vi "Single-Loop Queued State Machine.vi"() -> ()   [LabVIEW 2020]
uses:
  VIPackages/Custom Packages/Source LV2020-32b/SM Templates/StateMachine - AppData--cluster.ctl
panel:
  in  "Exit":bool
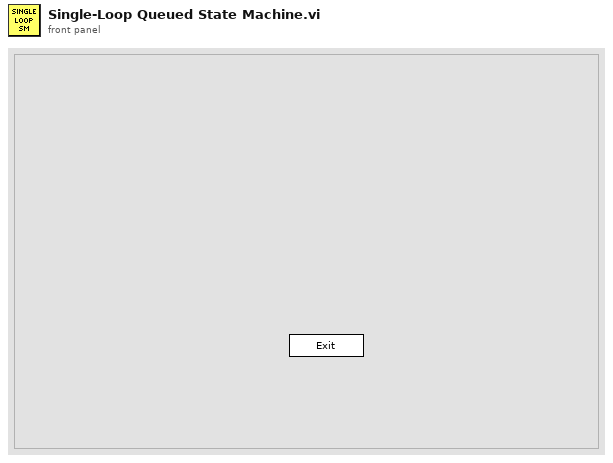
[diagram p1: front panel]
types:
  T1 = typedef "StateMachine - AppData--cluster.ctl" = cluster{"Core":cluster{"Current VI Reference":refnum<vi>, "Close Panel on Exit?":bool}, "Your Boolean data":bool, "Your string data":string}
  T2 = enum32{"invalid app kind", "Development System", "Run Time System", "Student Edition", "Embedded LabVIEW", "Evaluation", "Custom"}
  T3 = enum32{"Invalid", "Standard", "Closed", "Hidden", "Minimized", "Maximized"}
  T4 = cluster{"Current VI Reference":refnum<vi>, "Close Panel on Exit?":bool}
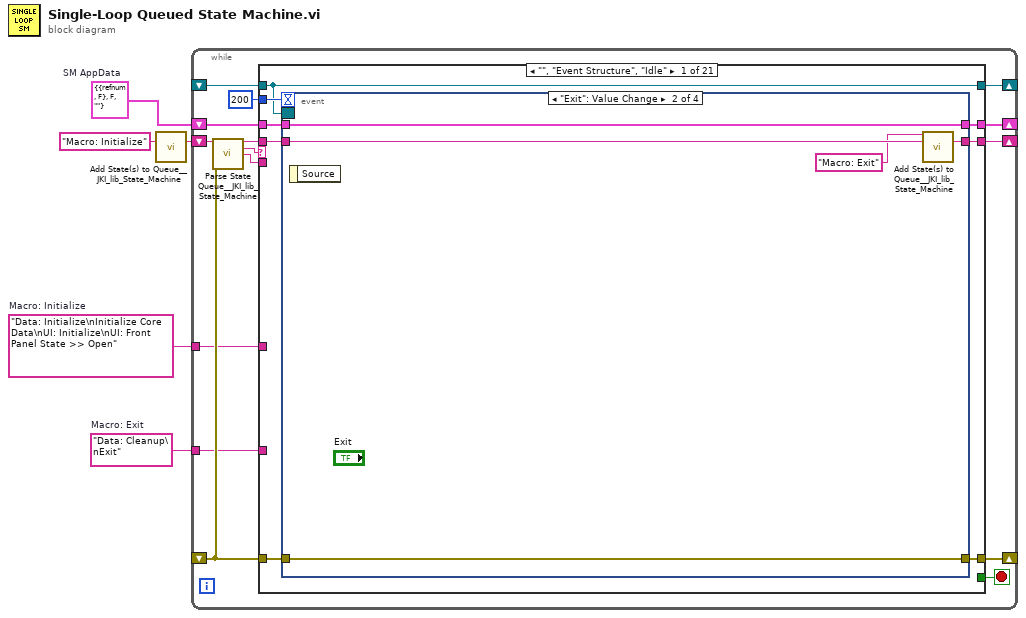
[diagram p0: block diagram]
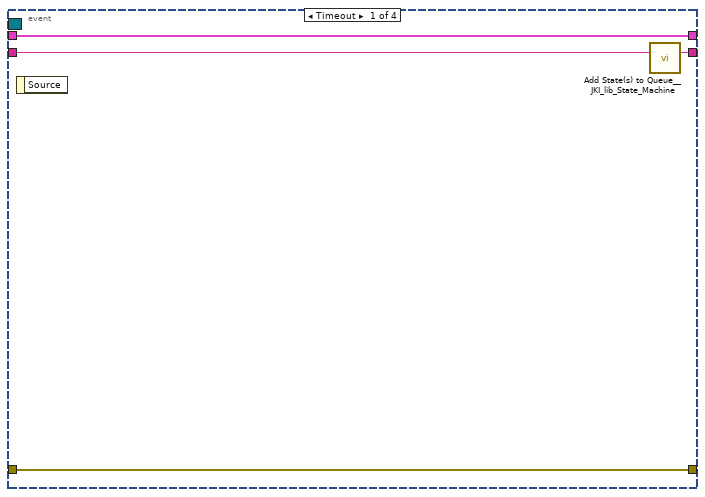
[diagram p2: hidden frame]
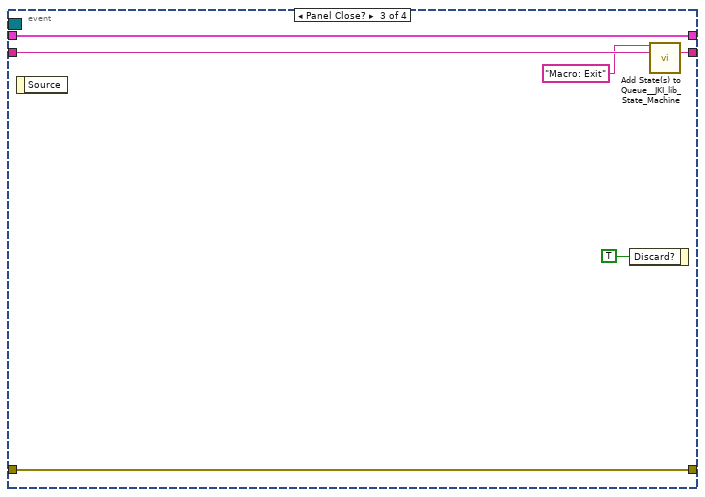
[diagram p3: hidden frame]
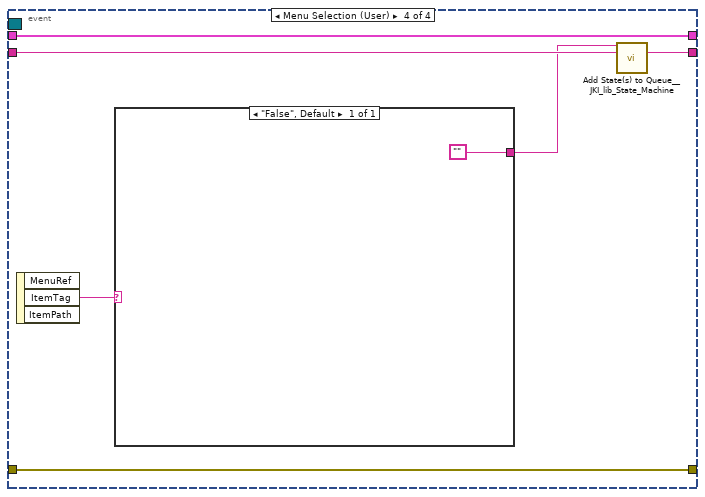
[diagram p4: hidden frame]
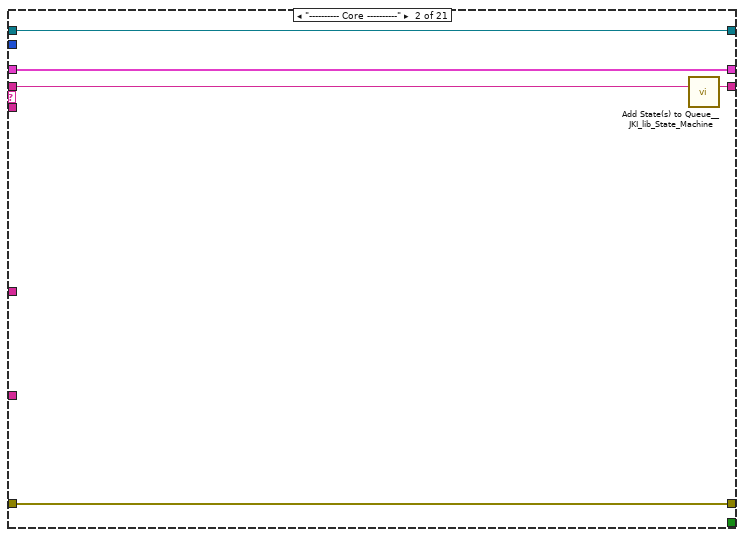
[diagram p5: hidden frame]
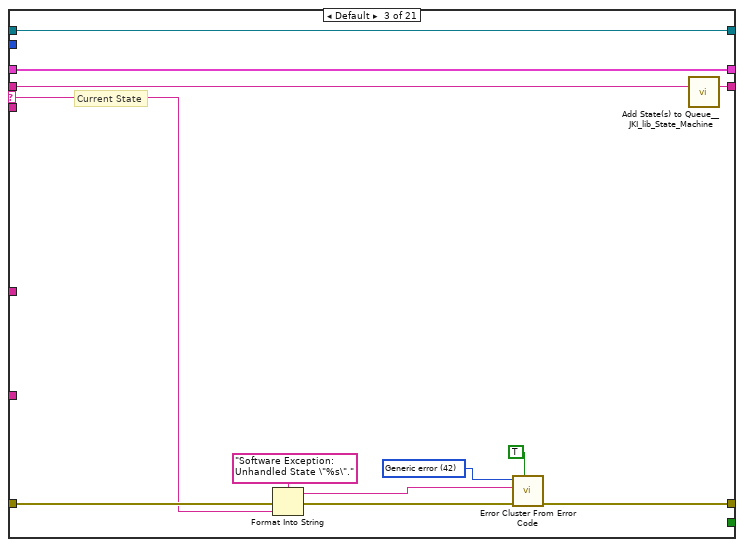
[diagram p6: hidden frame]
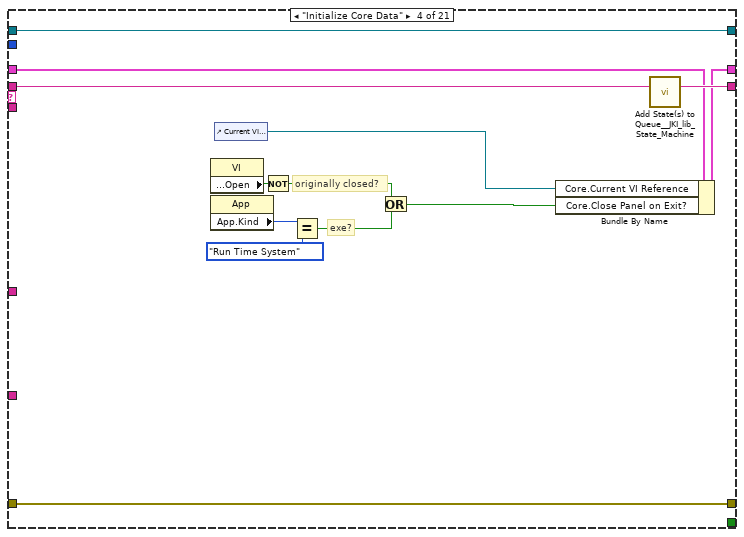
[diagram p7: hidden frame]
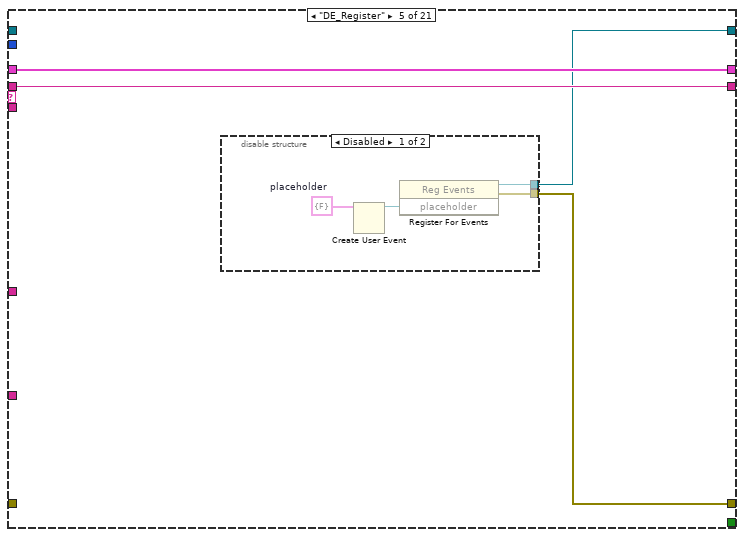
[diagram p8: hidden frame]
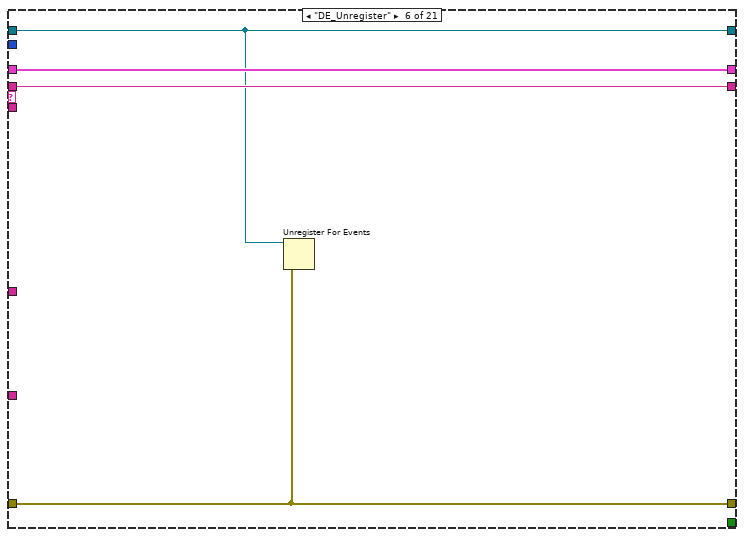
[diagram p10: hidden frame]
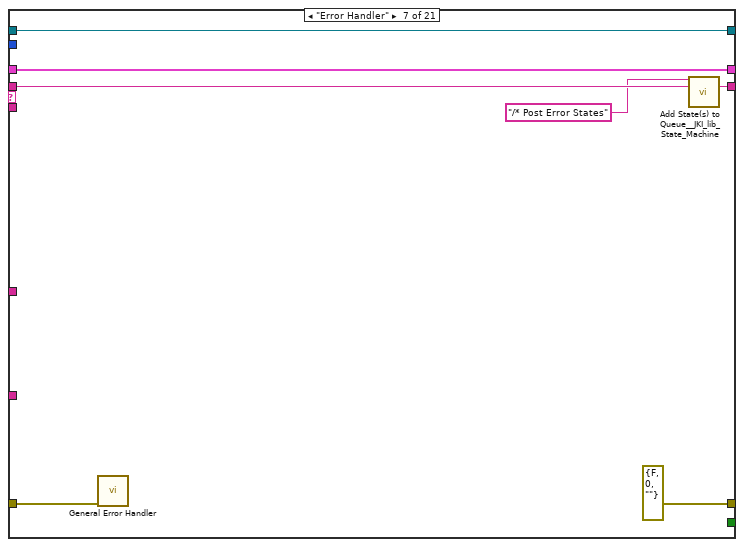
[diagram p11: hidden frame]
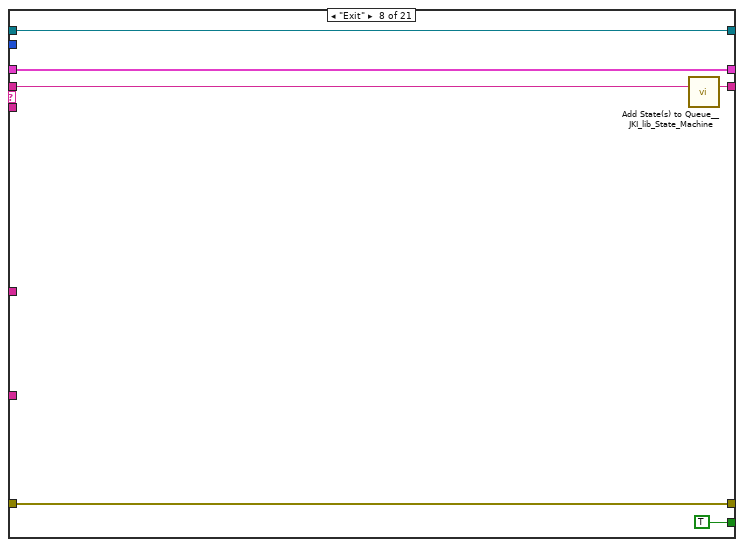
[diagram p12: hidden frame]
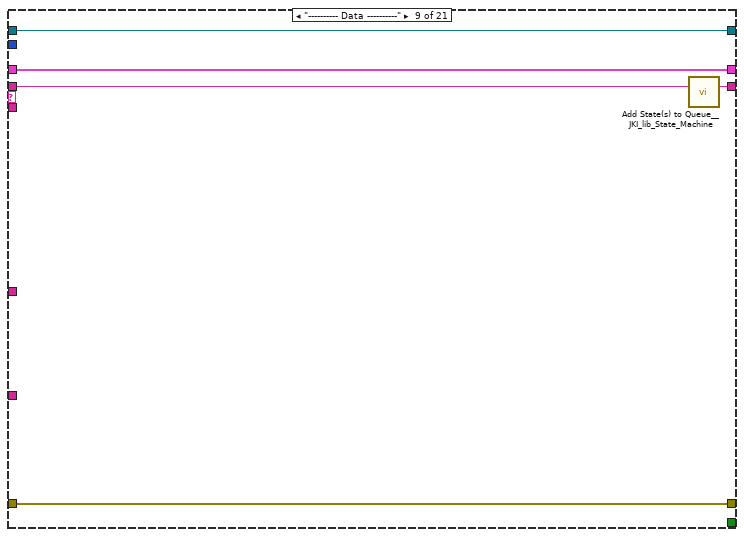
[diagram p13: hidden frame]
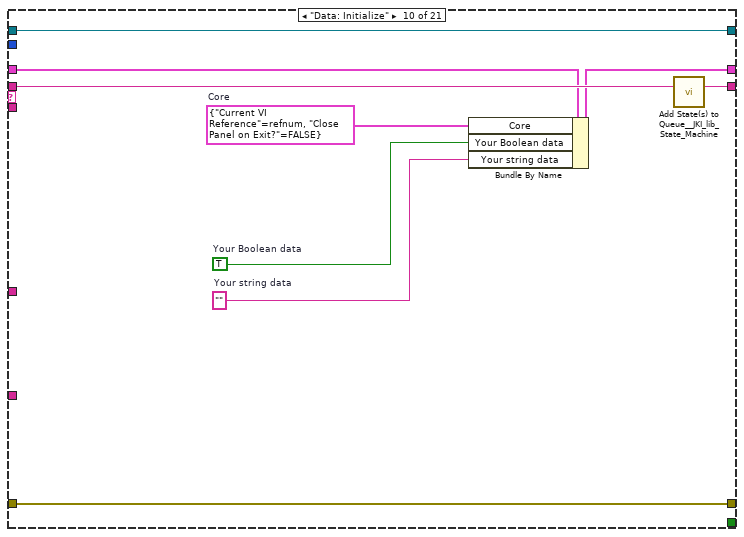
[diagram p14: hidden frame]
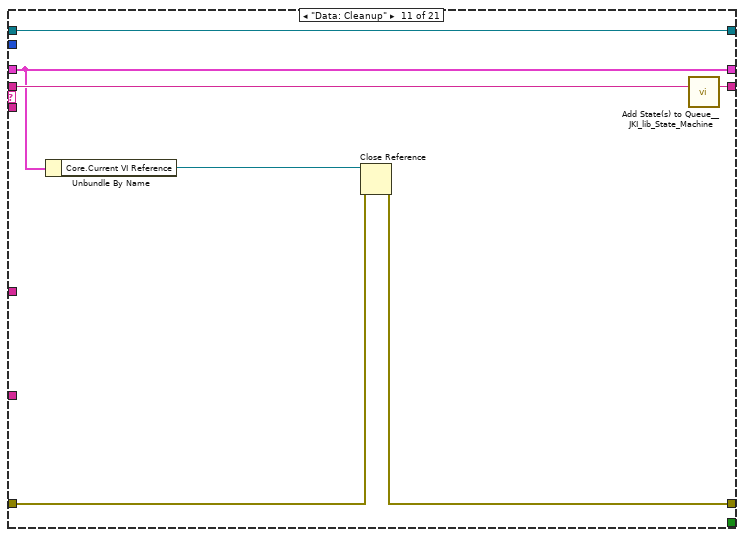
[diagram p15: hidden frame]
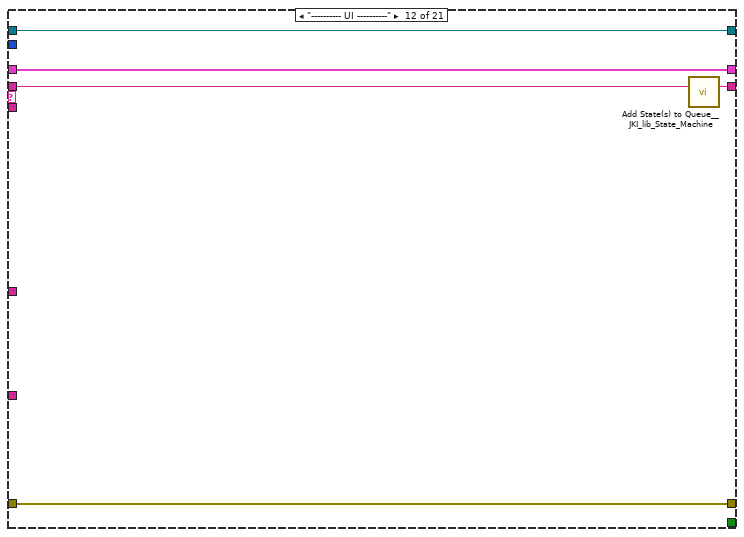
[diagram p16: hidden frame]
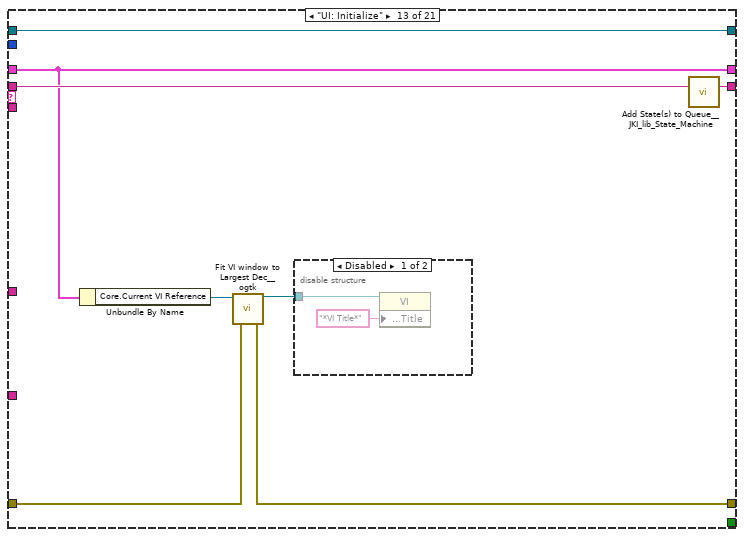
[diagram p17: hidden frame]
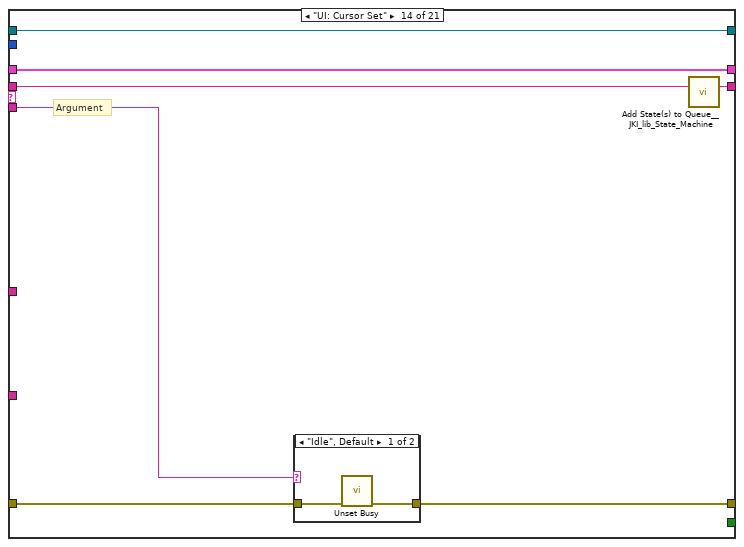
[diagram p19: hidden frame]
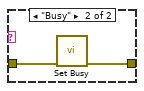
[diagram p20: hidden frame]
diagram:
  w1 = "Data: Cleanup\nExit"  # Macro: Exit
  w2 = "Data: Initialize\nInitialize Core Data\nUI: Initialize\nUI: Front Panel State >> Open"  # Macro: Initialize
  w3 = T1 {"Core"={"Current VI Reference"=refnum, "Close Panel on Exit?"=FALSE}, "Your Boolean data"=FALSE, "Your string data"=""}  # SM AppData
  n1 = call <vilib>:"Add State(s) to Queue__JKI_lib_State_Machine.vi"("State(s) in (\"\")"="Macro: Initialize") -> ("States Out"=w5:string)  [unwired: 14 in]
  n2 = while {
    shift-right: [w13] -> _
    shift-left: w3 -> [w12]
    shift-right: [w16] -> _
    shift-left: _ -> [w11]
    shift-right: [w15] -> _
    shift-left: w5 -> [w17]
    shift-right: [w10] -> _
    shift-left: _ -> [w9]
    tunnel: w2 -> [w7]
    tunnel: w1 -> [w6]
    stop <- w14 stop-if-true
    n3 = call <vilib>:"Parse State Queue__JKI_lib_State_Machine.vi"("State Queue"=w17, "Error In (no error)"=w11) -> ("Remaining States"=w19:string, "Current State"=w20:string, "Arguments"=w18:string)  [unwired: 11 in]
    n4 = case shown="\"\", \"Event Structure\", \"Idle\"" w20 {
      selector: w20 -> [_ _ w57 _ _ _ _ _ _ _ _ _ _ _ _ _ _ _ _ _ _]
      tunnel: w19 -> [w28 w55 w61 w80 w84 w92 w99 w105 w110 w119 w126 w131 w139 w148 w160 w187 w193 w204 w209 w220 w225]
      tunnel: w18 -> [_ _ _ _ _ _ _ _ _ _ _ _ _ w143 w154 _ _ _ _ w210 _]
      tunnel: w12 -> [w26 w52 w59 w71 w83 w91 w96 w103 w107 w113 w121 w128 w134 w146 w156 w184 w190 w201 w206 w218 w222]
      tunnel: [w25 w53 w63 w77 w81 w89 errorcluster {"status"=FALSE, "code"=0, "source"=""} ("error out") w102 w108 w117 w122 w129 w135 w144 w157 w185 w191 w202 w207 w211 w223] -> w16
      tunnel: w11 -> [w24 w53 w62 w77 _ w89 w95 w102 w108 w117 w123 w129 w136 w145 w158 w185 w191 w202 w207 w212 w223]
      tunnel: [w27 w54 w60 w79 w84 w92 w98 w104 w109 w118 w125 w130 w138 w147 w159 w186 w192 w203 w208 w219 w224] -> w15
      tunnel: [_ _ _ _ _ _ _ TRUE _ _ _ _ _ _ _ _ _ _ _ _ _] -> w14
      tunnel: [w23 w52 w59 w78 w83 w91 w96 w103 w107 w112 w121 w128 w134 w146 w156 w184 w190 w201 w206 w218 w222] -> w13
      tunnel: [w21 w51 w56 w68 w82 w90 w93 w100 w106 w111 w120 w127 w137 w142 w153 w183 w189 w195 w205 w217 w221] -> w10
      tunnel: w9 -> [w21 w51 w56 w68 _ w90 w93 w100 w106 w111 w120 w127 w137 w142 w153 w183 w189 w195 w205 w217 w221]
      tunnel: 200 ("Timeout") -> [w22 _ _ _ _ _ _ _ _ _ _ _ _ _ _ _ _ _ _ _ _]
      tunnel: w7 -> [_ _ _ _ _ _ _ _ _ _ _ _ _ _ _ _ w188 _ _ _ _]
      tunnel: w6 -> [_ _ _ _ _ _ _ _ _ _ _ _ _ _ _ _ _ w194 _ _ _]
      frame "", "Event Structure", "Idle" {
        n5 = event shown="[1] \"Exit\": Value Change" {
          selector: w21 -> [_ _ _ _]
          dyn-events: _ -> [_ _ _ _]
          timeout: w22 -> [_ _ _ _]
          tunnel: w28 -> [w32 w37 w43 w46]
          tunnel: [w31 w36 w42 w45] -> w27
          tunnel: w26 -> [w29 w34 w40 w48]
          tunnel: [w30 w35 w41 w49] -> w25
          tunnel: w24 -> [w30 w35 w41 w49]
          tunnel: [w29 w34 w40 w48] -> w23
          event Timeout {
            n6 = event-data() -> ()  [unwired: 1 in, 1 out]
            n7 = call <vilib>:"Add State(s) to Queue__JKI_lib_State_Machine.vi"("State(s) in (\"\")"=w32) -> ("States Out"=w31:string)  [unwired: 14 in]
          }
          event "Exit": Value Change {
            n8 = event-data() -> ()  [unwired: 1 in, 1 out]
            n9 = call <vilib>:"Add State(s) to Queue__JKI_lib_State_Machine.vi"("State(s) in Front (\"\")"="Macro: Exit", "State(s) in (\"\")"=w37) -> ("States Out"=w36:string)  [unwired: 13 in]
          }
          event Panel Close? {
            n10 = event-data() -> ()  [unwired: 1 in, 1 out]
            n11 = event-data("Discard?"=TRUE) -> ()  [unwired: 1 in, 1 out]
            n12 = call <vilib>:"Add State(s) to Queue__JKI_lib_State_Machine.vi"("State(s) in Front (\"\")"="Macro: Exit", "State(s) in (\"\")"=w43) -> ("States Out"=w42:string)  [unwired: 13 in]
          }
          event Menu Selection (User) {
            n13 = event-data() -> ("ItemTag"=w47:string)  [unwired: 1 in, 2 out]
            n14 = case shown="\"False\", Default" w47 {
              tunnel: [""] -> w44
              frame "False", Default {
              }
            }
            n15 = call <vilib>:"Add State(s) to Queue__JKI_lib_State_Machine.vi"("State(s) in Front (\"\")"=w44, "State(s) in (\"\")"=w46) -> ("States Out"=w45:string)  [unwired: 13 in]
          }
        }
      }
      frame "---------- Core ----------" {
        n16 = call <vilib>:"Add State(s) to Queue__JKI_lib_State_Machine.vi"("State(s) in (\"\")"=w55) -> ("States Out"=w54:string)  [unwired: 14 in]
      }
      frame Default {
        w66 = 42 items=["No error", "Argument error", "Memory is full", "Out of zone", "End of file", "File already open", "Generic file I/O error", "File not found", "File permission error", "Disk is full", "Duplicate path", "Too many files open", "System feature not enabled", "Resource file not found", "Cannot add resource", "Resource not found", "Image not found", "Image memory error", "Pen does not exist", "Config type invalid", "Config token not found", "Config parse error", "Config memory error", "Bad external code format", "Bad external code offset", "External code not present", "Null window", "Destroy window error", "Null menu", "Print aborted", "Bad print record", "Print driver error", "Windows error during printing", "Memory error during printing", "Print dialog error", "Generic print error", "Invalid device refnum", "Device not found", "Device parameter error", "Device unit error", "Cannot open device", "Device call aborted", "Generic error", "Cancelled by user", "Object ID too low", "Object ID too high", "Object not in heap", "Unknown heap", "Unknown object (invalid DefProc)", "Unknown object (DefProc not in table)", "Message out of range", "Invalid (null) method", "Unknown message", "Manager call not supported", "Bad address", "Network operation in progress", "Network operation timed out", "Connection is busy", "Network attribute not supported", "Network error", "Address in use", "System out of memory", "Connection aborted", "Connection refused", "Not connected", "Already connected", "Connection closed", "Initialization error (interapplication manager)", "Bad occurrence", "Wait on unbound occurrence handler", "Occurrence queue overflow", "Datalog type conflict", "Unused", "Unrecognized type (interapplication manager)", "Memory corrupt", "Failed to make temporary DLL", "Old CIN version", "Drag socket not found", "Failed to load drop-object", "Failed to register OLE object", "Failed to release OLE object", "Format specifier type mismatch", "Unknown format specifier", "Too few format specifiers", "Too many format specifiers", "Scan failed", "Newer CIN version", "Error converting to variant", "Runtime menu error", "Password tampered", "Variant attribute not found", "Incompatible variant data type", "Event data is not available", "Event Store is not present", "Occurrence is not found", "Event Queue is not created", "Event info is not available", "Refnum passed is NULL", "Error retrieving Class GUID", "Error retrieving CoClass GUID", "Error retrieving TypeLib GUID.", "Bad built application magic bytes.", "Specific driver is different from the specific driver associated with the Logical Name.", "There is no session opened to the class driver.", "Max Error", "MAX - Error with config objects", "MAX - Error loading configuration", "MAX - Group not supported"]
        # "Current State"
        n17 = Format Into String(format string="Software Exception: Unhandled State \"%s\"." ("message"), error in=w62, w57) -> (resulting string=w65:string, error out=w64:errorcluster)  [unwired: 1 in]
        n18 = call <vilib>:"Error Cluster From Error Code.vi"("show call chain? (False)"=TRUE, "error in (no error)"=w64, "error message (\"\")"=w65, "error code (0)"=w66) -> ("error out"=w63:errorcluster)  [unwired: 5 in]
        n19 = call <vilib>:"Add State(s) to Queue__JKI_lib_State_Machine.vi"("State(s) in (\"\")"=w61) -> ("States Out"=w60:string)  [unwired: 14 in]
      }
      frame "Initialize Core Data" {
        # "originally closed?"
        # "exe?"
        n20 = property class="VI"() -> ("Front Panel.Open"=w76:bool)  [unwired: 2 in, 2 out]
        n21 = property class="App"() -> ("App.Kind"=w75:T2)  [unwired: 2 in, 2 out]
        n22 = control-ref of="Current VI Reference"() -> (w69:refnum<vi>)
        n23 = Not(x=w76) -> (.not. x?=w73:bool)
        n24 = Equal?(x=w75, y=T2."Run Time System" ("Application:Kind")) -> (x = y?=w72:bool)
        n25 = Or(x=w73, y=w72) -> (x .or. y?=w70:bool)
        n26 = Bundle By Name(cluster=w71, "Core.Current VI Reference"=w69, "Core.Close Panel on Exit?"=w70) -> (w78:T1)
        n27 = call <vilib>:"Add State(s) to Queue__JKI_lib_State_Machine.vi"("State(s) in (\"\")"=w80) -> ("States Out"=w79:string)  [unwired: 14 in]
      }
      frame "DE_Register" {
        n28 = disable-structure shown="Disabled" {
          disable-tunnel: [w88 _] -> w82
          disable-tunnel: [w87 _] -> w81
          frame Disabled {
            w86 = cluster{bool} {FALSE}  # placeholder
            n29 = Create User Event(user event datatype=w86) -> (user event=w85:refnum<user-event>)  [unwired: 1 in, 1 out]
            n30 = register-events(w85) -> (reference out=w88:refnum<event-registration>, error out=w87:errorcluster)  [unwired: 2 in]
          }
          frame Enabled {
          }
        }
      }
      frame "DE_Unregister" {
        n31 = Unregister For Events(event registration refnum=w90, error in=w89) -> ()  [unwired: 1 out]
      }
      frame "Error Handler" {
        n32 = call <vilib>:"General Error Handler.vi"("error in (no error)"=w95) -> ()  [unwired: 10 in, 5 out]
        n33 = call <vilib>:"Add State(s) to Queue__JKI_lib_State_Machine.vi"("State(s) in Front (\"\")"="/* Post Error States", "State(s) in (\"\")"=w99) -> ("States Out"=w98:string)  [unwired: 13 in]
      }
      frame "Exit" {
        n34 = call <vilib>:"Add State(s) to Queue__JKI_lib_State_Machine.vi"("State(s) in (\"\")"=w105) -> ("States Out"=w104:string)  [unwired: 14 in]
      }
      frame "---------- Data ----------" {
        n35 = call <vilib>:"Add State(s) to Queue__JKI_lib_State_Machine.vi"("State(s) in (\"\")"=w110) -> ("States Out"=w109:string)  [unwired: 14 in]
      }
      frame "Data: Initialize" {
        w114 = T4 {"Current VI Reference"=refnum, "Close Panel on Exit?"=FALSE}  # Core
        w116 = TRUE  # Your Boolean data
        w115 = ""  # Your string data
        n36 = Bundle By Name(cluster=w113, "Core"=w114, "Your Boolean data"=w116, "Your string data"=w115) -> (w112:T1)
        n37 = call <vilib>:"Add State(s) to Queue__JKI_lib_State_Machine.vi"("State(s) in (\"\")"=w119) -> ("States Out"=w118:string)  [unwired: 14 in]
      }
      frame "Data: Cleanup" {
        n38 = Unbundle By Name(w121) -> ("Core.Current VI Reference"=w124:refnum<vi>)
        n39 = Close Reference(reference=w124, error in (no error)=w123) -> (error out=w122:errorcluster)
        n40 = call <vilib>:"Add State(s) to Queue__JKI_lib_State_Machine.vi"("State(s) in (\"\")"=w126) -> ("States Out"=w125:string)  [unwired: 14 in]
      }
      frame "---------- UI ----------" {
        n41 = call <vilib>:"Add State(s) to Queue__JKI_lib_State_Machine.vi"("State(s) in (\"\")"=w131) -> ("States Out"=w130:string)  [unwired: 14 in]
      }
      frame "UI: Initialize" {
        n42 = Unbundle By Name(w134) -> ("Core.Current VI Reference"=w133:refnum<vi>)
        n43 = call <userlib>:"Fit VI window to Largest Dec__ogtk.vi"("error in (no error)"=w136, "VI Ref (calling VI)"=w133) -> ("error out"=w135:errorcluster, "dup VI Ref"=w132:refnum<vi>)  [unwired: 4 in]
        n44 = disable-structure shown="Disabled" {
          disable-tunnel: w132 -> [w141 _]
          frame Disabled {
            n45 = property class="VI"(reference=w141, "Front Panel.Title"="*VI Title*" ("Front Panel Window:Title")) -> ()  [unwired: 1 in, 2 out]
          }
          frame Enabled {
          }
        }
        n46 = call <vilib>:"Add State(s) to Queue__JKI_lib_State_Machine.vi"("State(s) in (\"\")"=w139) -> ("States Out"=w138:string)  [unwired: 14 in]
      }
      frame "UI: Cursor Set" {
        # "Argument"
        n47 = case shown="\"Idle\", Default" w143 {
          tunnel: w145 -> [w150 w152]
          tunnel: [w149 w151] -> w144
          frame "Idle", Default {
            n48 = call <vilib>:"Unset Busy.vi"("error in (no error)"=w150) -> ("error out"=w149:errorcluster)  [unwired: 10 in]
          }
          frame "Busy" {
            n49 = call <vilib>:"Set Busy.vi"("error in (no error)"=w152) -> ("error out"=w151:errorcluster)  [unwired: 9 in, 1 out]
          }
        }
        n50 = call <vilib>:"Add State(s) to Queue__JKI_lib_State_Machine.vi"("State(s) in (\"\")"=w148) -> ("States Out"=w147:string)  [unwired: 14 in]
      }
      frame "UI: Front Panel State" {
        # "Argument"
        n51 = Unbundle By Name(w156) -> ("Core.Current VI Reference"=w155:refnum<vi>)
        n52 = case shown="\"Close\"" w154 {
          tunnel: w158 -> [w164 w177]
          tunnel: [w166 w178] -> w157
          tunnel: w155 -> [w165 w175]
          frame "Open", Default {
            n53 = property class="VI"(reference=w165, error in=w164) -> (reference out=w162:refnum<vi>, error out=w163:errorcluster, "Front Panel.Open"=w161:bool)
            n54 = case shown="False" w161 {
              tunnel: [w169 w172] -> w166
              tunnel: w163 -> [w168 w172]
              tunnel: w162 -> [w167 _]
              frame False {
                n55 = invoke class="VI" method="FP.Open"(reference=w167, error in=w168, "Activate"=TRUE, "State"=T3."Standard") -> (error out=w169:errorcluster)  [unwired: 1 in, 4 out]
              }
              frame True {
              }
            }
          }
          frame "Close" {
            n56 = property class="VI"(reference=w175, error in=w177) -> (reference out=w174:refnum<vi>, error out=w176:errorcluster, "Front Panel.Open"=w173:bool)
            n57 = case shown="True" w173 {
              tunnel: [w179 w182] -> w178
              tunnel: w176 -> [w179 w181]
              tunnel: w174 -> [_ w180]
              frame False {
              }
              frame True {
                n58 = invoke class="VI" method="FP.Close"(reference=w180, error in=w181) -> (error out=w182:errorcluster)  [unwired: 1 in, 2 out]
              }
            }
          }
        }
        n59 = call <vilib>:"Add State(s) to Queue__JKI_lib_State_Machine.vi"("State(s) in (\"\")"=w160) -> ("States Out"=w159:string)  [unwired: 14 in]
      }
      frame "---------- Macro ----------" {
        n60 = call <vilib>:"Add State(s) to Queue__JKI_lib_State_Machine.vi"("State(s) in (\"\")"=w187) -> ("States Out"=w186:string)  [unwired: 14 in]
      }
      frame "Macro: Initialize" {
        n61 = call <vilib>:"Add State(s) to Queue__JKI_lib_State_Machine.vi"("State(s) in Front (\"\")"=w188, "State(s) in (\"\")"=w193) -> ("States Out"=w192:string)  [unwired: 13 in]
      }
      frame "Macro: Exit" {
        n62 = Unbundle By Name(w201) -> ("Core.Close Panel on Exit?"=w200:bool)
        n63 = Select(t="UI: Front Panel State >> Close", s=w200, f="") -> (s? t:f=w197:string)
        n64 = call <vilib>:"Add State(s) to Queue__JKI_lib_State_Machine.vi"("State(s) in (\"\")"=w197, "State(s) at Back (\"\")"=w194) -> ("States Out"=w196:string)  [unwired: 13 in]
        n65 = call <vilib>:"Add State(s) to Queue__JKI_lib_State_Machine.vi"("State(s) in Front (\"\")"=w196, "State(s) in (\"\")"=w204) -> ("States Out"=w203:string)  [unwired: 13 in]
      }
      frame "---------- Action ----------" {
        n66 = call <vilib>:"Add State(s) to Queue__JKI_lib_State_Machine.vi"("State(s) in (\"\")"=w209) -> ("States Out"=w208:string)  [unwired: 14 in]
      }
      frame "Action: Wait" {
        n67 = Scan From String(format string="%d", input string=w210, error in=w212, default 1=u32 0) -> (error out=w216:errorcluster, output 1=w215:u32)  [unwired: 1 in, 2 out]
        n68 = call <userlib>:"Wait (ms)__ogtk.vi"("error in (no error)"=w216, "milliseconds to wait"=w215) -> ("error out"=w211:errorcluster)  [unwired: 8 in, 1 out]
        n69 = call <vilib>:"Add State(s) to Queue__JKI_lib_State_Machine.vi"("State(s) in (\"\")"=w220) -> ("States Out"=w219:string)  [unwired: 14 in]
      }
      frame "Action: 2" {
        n70 = call <vilib>:"Add State(s) to Queue__JKI_lib_State_Machine.vi"("State(s) in (\"\")"=w225) -> ("States Out"=w224:string)  [unwired: 14 in]
      }
    }
  }
